vi "Handle Command.vi"(8 "error in (no error)":errorcluster, 9 "Data":variant, 10 "Command":string, 11 "Inst.AH2500 in":refnum<class "Inst.AH2500.lvclass">) -> (0 "error out":errorcluster, 1 "Processed Data":variant, 2 "Command":string, 3 "Inst.AH2500 out":refnum<class "Inst.AH2500.lvclass">)   [LabVIEW 2019, in "Inst.AH2500.lvclass"]
uses:
  Inst.AH2500.lvclass
  Typedefs/Inst.AH2500.getAll--Cluster.ctl
  Inst.AH2500.lvclass/Inst.AH2500.ctl
  <userlib>/LevyLab/Instrument Framework/Instrument Types/VSource/Instrument.VSource.lvclass
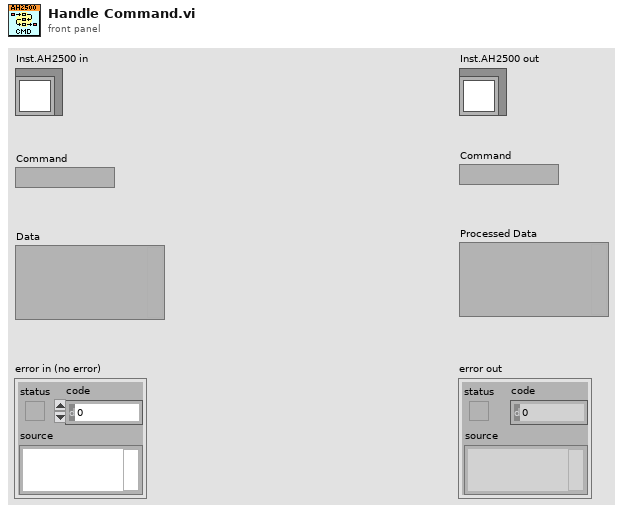
[diagram p1: front panel]
types:
  T1 = typedef "Inst.AH2500.lvclass/Inst.AH2500.getAll--Cluster.ctl" = cluster{"capacitance (pF)":dbl, "loss (nS)":dbl, "Vexc (V)":dbl}
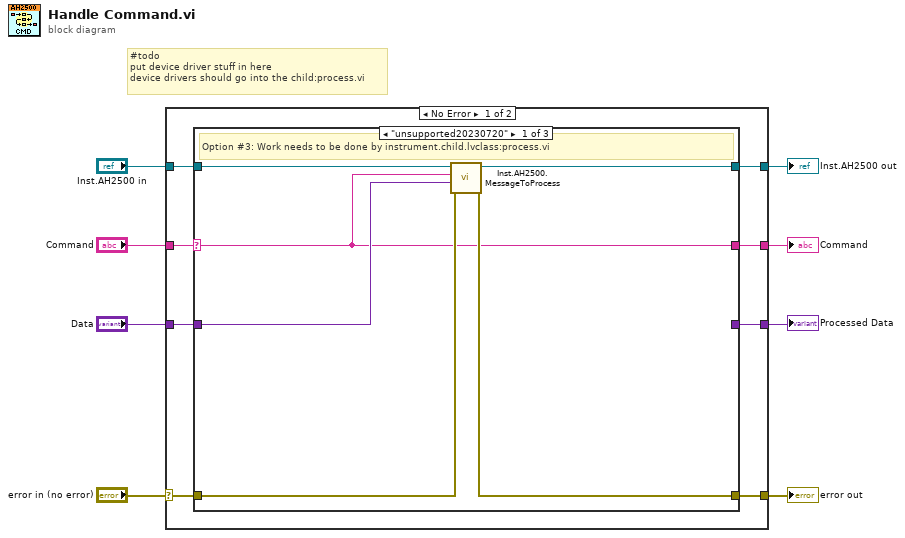
[diagram p0: block diagram]
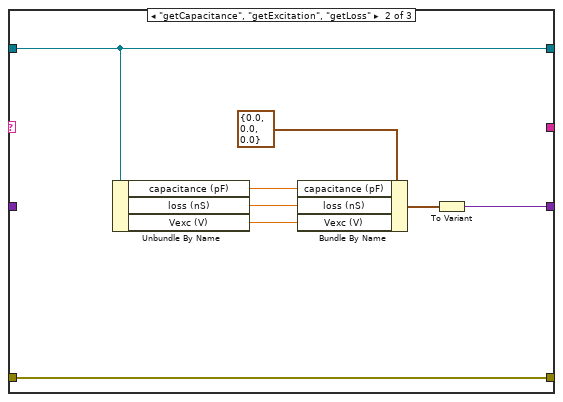
[diagram p2: hidden frame]
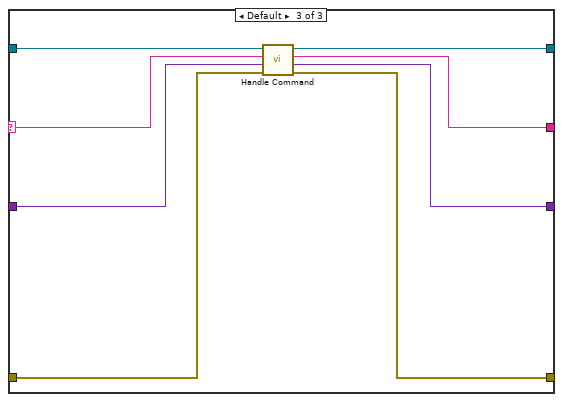
[diagram p3: hidden frame]
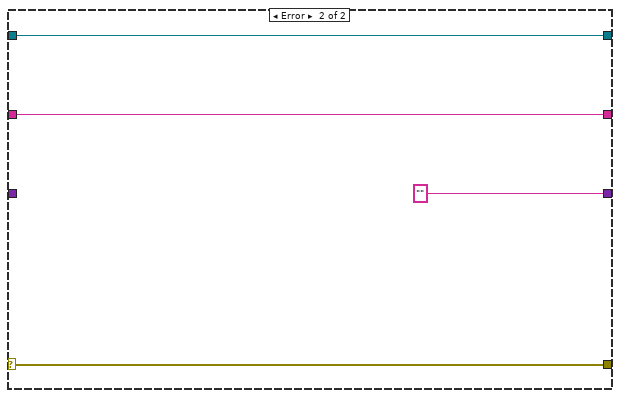
[diagram p4: hidden frame]
diagram:
  # "#todo\nput device driver stuff in here\ndevice drivers should go into the child:process.vi"
  n1 = case shown="No Error" "error in (no error)" {
    selector: "error in (no error)" -> [w10 w42]
    tunnel: [w12 w42] -> w6
    tunnel: [w14 w41] -> w5
    tunnel: "Inst.AH2500 in" -> [w15 w41]
    tunnel: "Command" -> [w16 w39]
    tunnel: [w13 "" ("String")] -> w3
    tunnel: "Data" -> [w9 _]
    tunnel: [w11 w39] -> w1
    frame No Error {
      n2 = case shown="\"unsupported20230720\"" w16 {
        selector: w16 -> [w17 _ w32]
        tunnel: w15 -> [w22 w30 w36]
        tunnel: [w21 w30 w33] -> w14
        tunnel: [_ w29 w35] -> w13
        tunnel: w10 -> [w20 w28 w37]
        tunnel: w9 -> [w18 _ w38]
        tunnel: [w19 w28 w34] -> w12
        tunnel: [w17 _ w31] -> w11
        frame "unsupported20230720" {
          # "Option #3: Work needs to be done by instrument.child.lvclass:process.vi"
          n3 = call "Inst.AH2500.MessageToProcess.vi"("error in (no error)"=w20, "Data"=w18, "Command"=w17, "Inst.AH2500 in"=w22) -> ("error out"=w19:errorcluster, "Inst.AH2500 out"=w21:refnum<class "Inst.AH2500.lvclass">)  [unwired: 6 in]
        }
        frame "getCapacitance", "getExcitation", "getLoss" {
          n4 = Unbundle By Name(w30) -> ("capacitance (pF)"=w26:dbl, "loss (nS)"=w24:dbl, "Vexc (V)"=w23:dbl)
          n5 = Bundle By Name(cluster=T1 {"capacitance (pF)"=0.0, "loss (nS)"=0.0, "Vexc (V)"=0.0} ("getAll"), "capacitance (pF)"=w26, "loss (nS)"=w24, "Vexc (V)"=w23) -> (w25:T1)
          n6 = To Variant(anything=w25) -> (Variant=w29:variant)
        }
        frame Default {
          n7 = call-parent "Handle Command.vi"("error in (no error)"=w37, "params in"=w38, "command"=w32, "Instrument in"=w36) -> ("error out"=w34:errorcluster, "processed data"=w35:variant, "command out"=w31:string, "Instrument out"=w33:refnum<class "Inst.AH2500.lvclass">)  [unwired: 4 in]
        }
      }
    }
    frame Error {
    }
  }
  "error out" <- w6
  "Inst.AH2500 out" <- w5
  "Command" <- w1
  "Processed Data" <- w3
